vi "Write clearErrorIsTrue.vi"(8 "error in (no error)":errorcluster, 10 "clearErrorIsTrue":bool, 11 "ApplicationHandler in":refnum<class "ApplicationHandler.lvclass">) -> (0 "error out":errorcluster, 3 "ApplicationHandler out":refnum<class "ApplicationHandler.lvclass">)   [LabVIEW 2013, in "ComponentData.lvlib" / "ApplicationHandler.lvclass"]
uses:
  <userlib>/Common/Component/common_application/RT/ComponentData/ApplicationHandler/ApplicationHandler.lvclass
  <userlib>/Common/Component/common_application/RT/ComponentData/ApplicationHandler/ApplicationHandler.lvclass/ApplicationHandler.ctl
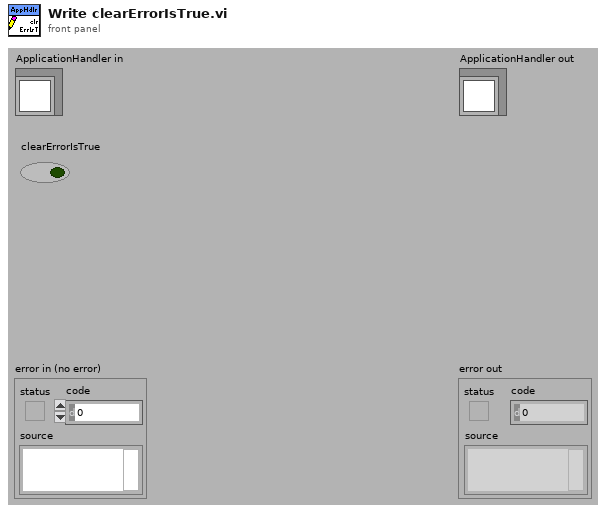
[diagram p1: front panel]
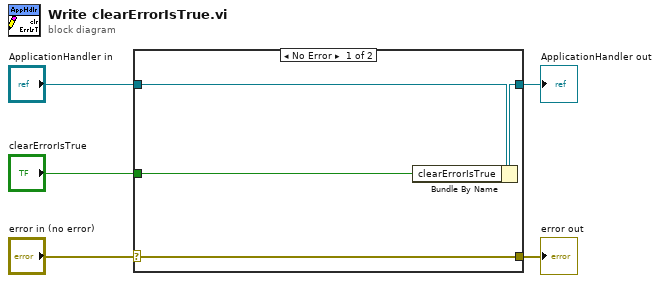
[diagram p0: block diagram]
diagram:
  n1 = case shown="No Error" "error in (no error)" {
    selector: "error in (no error)" -> [w9 w10]
    tunnel: [w9 w10] -> w4
    tunnel: [w7 w11] -> w2
    tunnel: "ApplicationHandler in" -> [w8 w11]
    tunnel: "clearErrorIsTrue" -> [w6 _]
    frame No Error {
      n2 = Bundle By Name(cluster=w8, "clearErrorIsTrue"=w6) -> (w7:refnum<class "ApplicationHandler.lvclass">)
    }
    frame Error {
    }
  }
  "error out" <- w4
  "ApplicationHandler out" <- w2
